vi "Measurement Logic.vi"() -> ()   [LabVIEW 2021, in "ImageStreamRendering.lvlib"]
uses:
  ImageStreamRendering.lvlib
  Measurement Configuration.ctl
  Measurement Results.ctl
  <vilib>/MeasurementLink/MeasurementLink Measurement Server/Measure Call Context/Measure Call Context.lvclass
  <vilib>/vision/driver/IMAQdx.llb/IMAQdx Camera Control Mode.ctl
  <vilib>/vision/driver/IMAQdx.llb/IMAQdx Acquisition Mode.ctl
  <vilib>/MeasurementLink/MeasurementLink Measurement Server/Measure Call Context/Accessor/Is Canceled.vi
  <vilib>/vision/driver/NI_Vision_Acquisition_Software.lvlib
panel:
  out "measure call context out":refnum<class "Measure Call Context.lvclass">
  in  "measure call context in":refnum<class "Measure Call Context.lvclass">
  out "measurement results":T1={"Image Data"="Empty", "Image Resolution"=[], "Image Pixels (U32)"=[], "Last Buffer Number"=0, "Image Acq time"=""}
  in  "measurement configuration":T2={"Camera name"="D:\\Avi\\_PRK5307.jpg", "Image Converison Type"="", "External Display"=FALSE}
  out "error out":errorcluster
  in  "error in":errorcluster
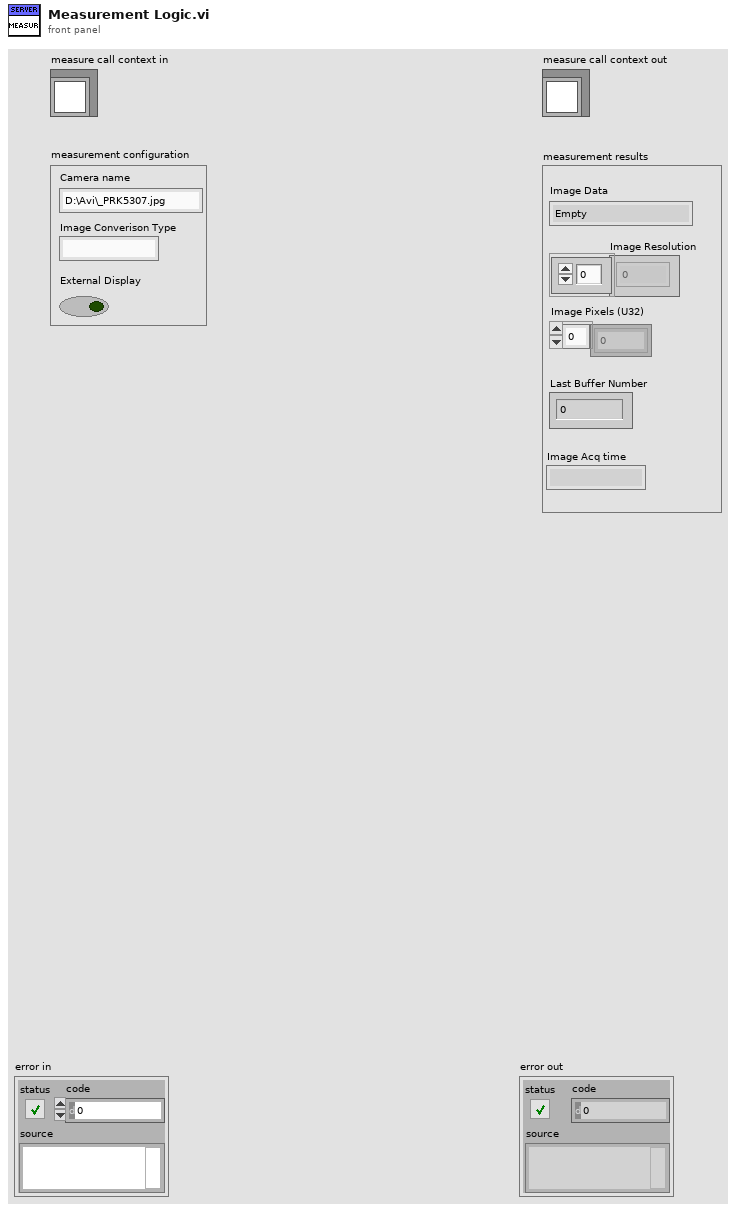
[diagram p1: front panel]
types:
  T1 = typedef "ImageStreamRendering.lvlib/Measurement Results.ctl" = cluster{"Image Data":string, "Image Resolution":i32[], "Image Pixels (U32)":u32[], "Last Buffer Number":u32, "Image Acq time":string}
  T2 = typedef "ImageStreamRendering.lvlib/Measurement Configuration.ctl" = cluster{"Camera name":string, "Image Converison Type":string, "External Display":bool}
  T3 = typedef "NI_Vision_Acquisition_Software.lvlib/IMAQdx Acquisition Mode.ctl" = enum32{"One Shot", "Continuous"}
  T4 = typedef "NI_Vision_Acquisition_Software.lvlib/IMAQdx Camera Control Mode.ctl" = enum32{"Controller", "Listener"}
  T5 = typedef "IMAQdx.ctl" = refnum<k21>
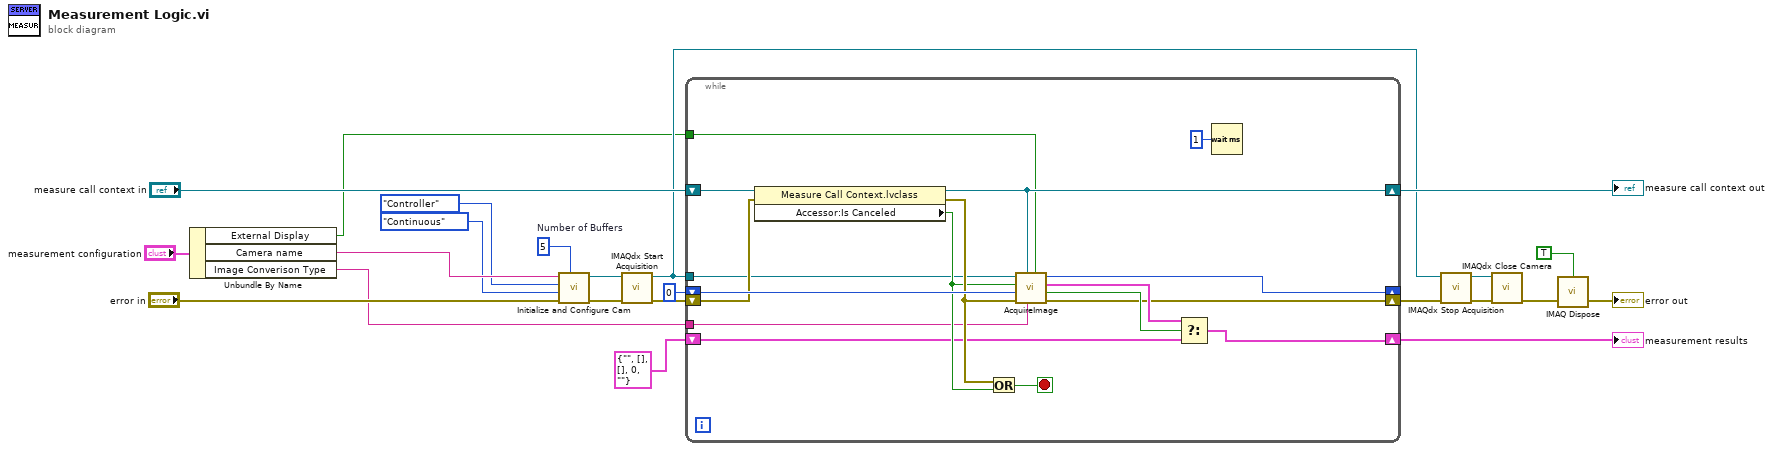
[diagram p0: block diagram]
diagram:
  w17 = u32 5  # Number of Buffers
  n1 = Unbundle By Name("measurement configuration") -> ("External Display"=w1:bool, "Camera name"=w22:string, "Image Converison Type"=w11:string)
  n2 = call "Initialize and Configure Cam.vi"("Number of Buffers"=w17, "error in"="error in", "Continuous?"=IMAQdx_Acquisition_Mode."Continuous", "Camera Control Mode"=IMAQdx_Camera_Control_Mode."Controller", "Camera name"=w22) -> ("error out"=w21:errorcluster, "camera session out"=w20:T5)  [unwired: 5 in]
  n3 = call <vilib>:"IMAQdx Start Acquisition.vi"("error in"=w21, "Session In"=w20) -> ("error out"=w13:errorcluster, "Session Out"=w7:T5)  [unwired: 8 in]
  n4 = while {
    shift-right: [w34] -> w14
    shift-left: "measure call context in" -> [w40]
    tunnel: w7 -> [w28]
    shift-right: [w27] -> _
    shift-left: u32 0 ("Buffer Number Out") -> [w39]
    tunnel: w11 -> [w35]
    shift-right: [w30] -> w9
    shift-left: T1 {"Image Data"="", "Image Resolution"=[], "Image Pixels (U32)"=[], "Last Buffer Number"=0, "Image Acq time"=""} ("Measurement Results") -> [w31]
    shift-right: [w26] -> w8
    shift-left: w13 -> [w38]
    tunnel: w1 -> [w24]
    stop <- w25 stop-if-true
    n5 = property class="Measure Call Context.lvclass"(reference=w40, error in=w38) -> (reference out=w34:refnum<class "Measure Call Context.lvclass">, error out=w37:errorcluster, "Accessor:Is Canceled"=w36:bool)
    n6 = Or(x=w37, y=w36) -> (x .or. y?=w25:bool)
    n7 = call "AcquireImage.vi"("External display"=w24, "Image Conversion"=w35, "measure call context in"=w34, "error in (no error)"=w37, "Buffer Number Out in"=w39, "Accessor:Is Canceled"=w36, "Refnum in"=w28) -> ("error out"=w26:errorcluster, "Valid Result"=w33:bool, "Measurement Results"=w32:T1, "Buffer Number Out out"=w27:u32)  [unwired: 1 in]
    n8 = Select(t=w32, s=w33, f=w31) -> (s? t:f=w30:T1)
    n9 = Wait (ms)(milliseconds to wait=u32 1) -> ()  [unwired: 1 out]
  }
  "measurement results" <- w9
  "measure call context out" <- w14
  n10 = call <vilib>:"IMAQdx Stop Acquisition.vi"("error in"=w8, "Session In"=w7) -> ("error out"=w5:errorcluster, "Session Out"=w6:T5)  [unwired: 8 in]
  n11 = call <vilib>:"IMAQdx Close Camera.vi"("error in"=w5, "Session In"=w6) -> ("error out"=w4:errorcluster)  [unwired: 9 in]
  n12 = call "IMAQ Dispose"("All Images? (No)"=TRUE, "error in (no error)"=w4) -> ("error out"=→"error out":errorcluster)  [unwired: 4 in]
